vi "RobotGoToCoord.vi"(1 "X/Y/a Target":T11, 2 "RobotDriveDevRef":T1={"DevStatus"={"status"=FALSE, "code"=0, "source"=""}, "Motors[]"=[], "Square Inputs"=FALSE, "Max Output"=1.0}) -> (0 "Done?":bool)   [LabVIEW 2014]
uses:
  <vilib>/Rock Robotics/WPI/RobotDrive/WPI_RobotDriveDevRef.ctl
  <vilib>/Rock Robotics/WPI/MotorControl/WPI_MotorControlDeviceRef.ctl
  <vilib>/Rock Robotics/WPI/MotorControl/WPI_MotorControlType.ctl
  <vilib>/Rock Robotics/SystemInterfaces/Typedef/FPGA_TypedefDigitalModule.ctl
  <vilib>/Rock Robotics/SystemInterfaces/DIO/FPGA_DIOPWMChannel.ctl
  <vilib>/Rock Robotics/WPI/PWM/WPI_PWMDeadband.ctl
  <vilib>/Rock Robotics/WPI/CAN/Jaguar/SubVIs/WPI_CANJaguar_ControlMode.ctl
  <vilib>/Rock Robotics/WPI/CAN/TalonSRX/WPI_CANTalonSRX_APIControlMode.ctl
  <vilib>/Rock Robotics/WPI/PWM/WPI_PWMTransform_ConPane.ctl
  Robot Global Data.vi
  <vilib>/express/express arith-compare/Formula/XNode/ExpressFormulaBlockNode.xnode
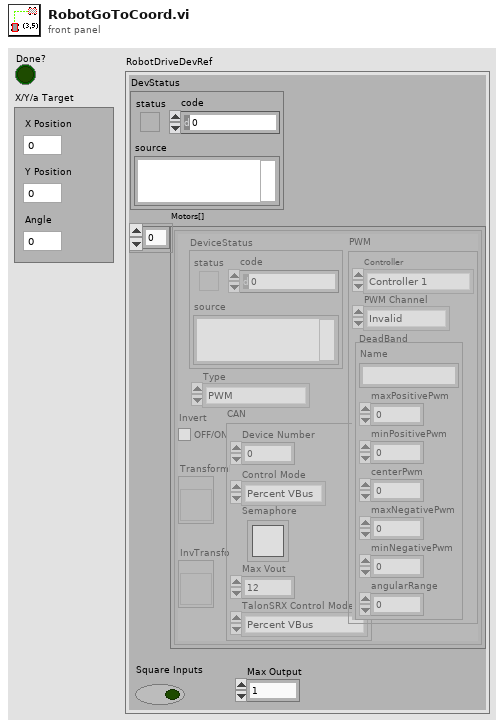
[diagram p1: front panel]
types:
  T1 = typedef "WPI_RobotDriveDevRef.ctl" = cluster{"DevStatus":errorcluster, "Motors[]":T2[], "Square Inputs":bool, "Max Output":dbl}
  T2 = typedef "WPI_MotorControlDeviceRef.ctl" = cluster{"DeviceStatus":errorcluster, "Type":T3, "PWM":cluster{"Controller":T4, "PWM Channel":T5, "DeadBand":T6}, "CAN":cluster{"Device Number":u8, "Control Mode":T7, "Semaphore":T8, "Max Vout":dbl, "TalonSRX Control Mode":T9}, "Invert":bool, "TransformRef":T10, "InvTransformRef":T10}
  T3 = typedef "WPI_MotorControlType.ctl" = enum16{"PWM", "CAN", "CANTalonSRX"}
  T4 = typedef "FPGA_TypedefDigitalModule.ctl" = enum16{"Controller 1"}
  T5 = typedef "FPGA_DIOPWMChannel.ctl" = enum8{"PWM 0", "PWM 1", "PWM 2", "PWM 3", "PWM 4", "PWM 5", "PWM 6", "PWM 7", "PWM 8", "PWM 9", "PWM MXP 0", "PWM MXP 1", "PWM MXP 2", "PWM MXP 3", "PWM MXP 4", "PWM MXP 5", "PWM MXP 6", "PWM MXP 7", "PWM MXP 8", "PWM MXP 9", "Invalid"}
  T6 = typedef "WPI_PWMDeadband.ctl" = cluster{"Name":string, "maxPositivePwm":i32, "minPositivePwm":i32, "centerPwm":i32, "maxNegativePwm":i32, "minNegativePwm":i32, "angularRange":u16}
  T7 = typedef "WPI_CANJaguar_ControlMode.ctl" = enum8{"Percent VBus", "Current", "Speed", "Position", "Voltage"}
  T8 = typedef "Semaphore RefNum" = refnum<k1>
  T9 = typedef "WPI_CANTalonSRX_APIControlMode.ctl" = enum8{"Percent VBus", "Speed", "Position", "Slave", "Unchanged / Invalid"}
  T10 = typedef "WPI_PWMTransform_ConPane.ctl" = refnum<vi>
  T11 = cluster{"X Position":dbl, "Y Position":dbl, "Angle":dbl}
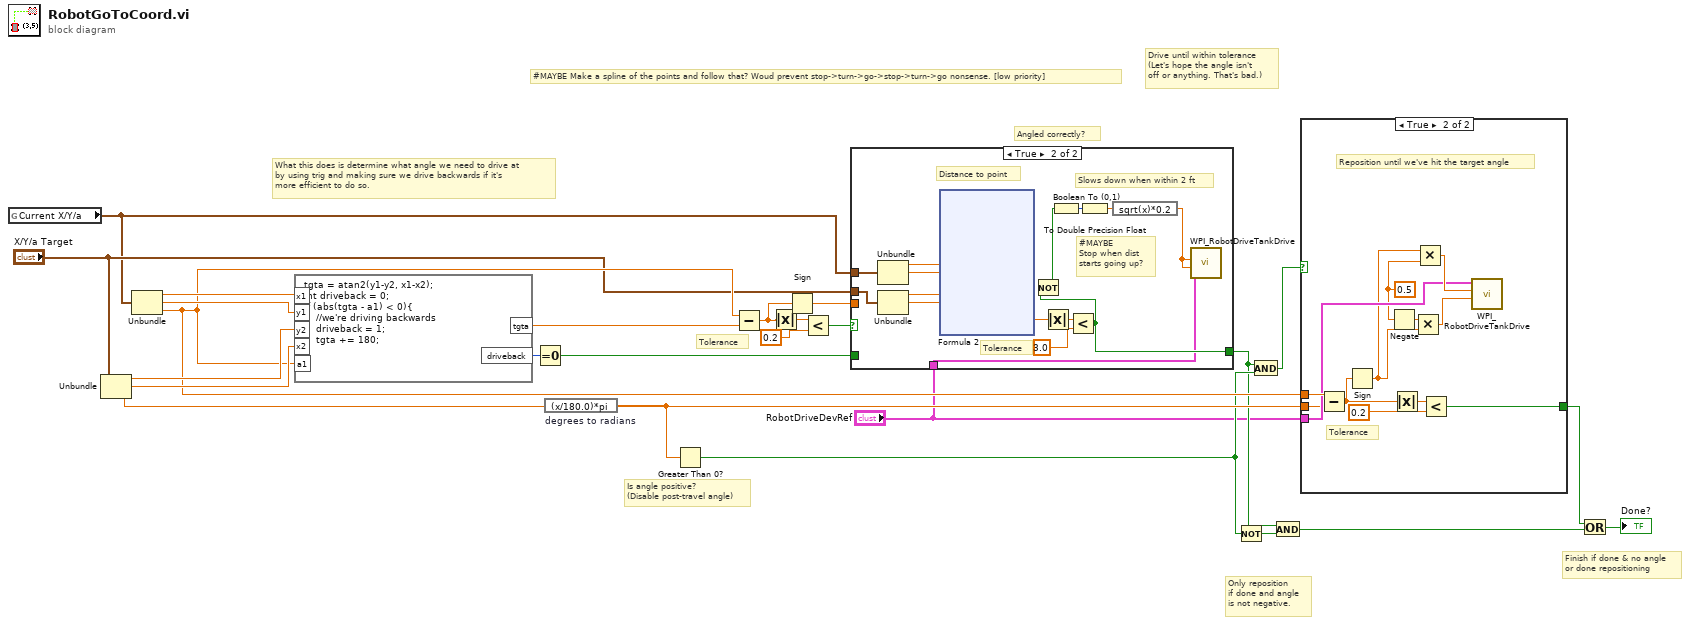
[diagram p0: block diagram]
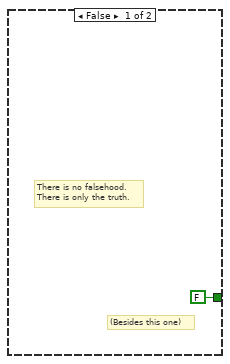
[diagram p2: hidden frame]
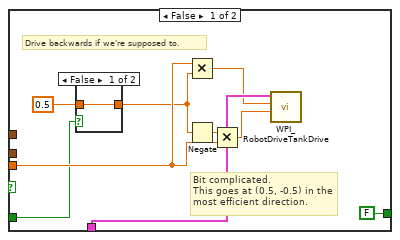
[diagram p3: hidden frame]
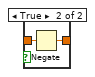
[diagram p4: hidden frame]
diagram:
  # "Drive until within tolerance\n(Let's hope the angle isn't\noff or anything. That's bad.)"
  # "What this does is determine what angle we need to drive at\nby using trig and making sure we drive backwards if it's\nmore efficient to do so."
  # "#MAYBE Make a spline of the points and follow that? Woud prevent stop->turn->go->stop->turn->go nonsense. [low priority]"
  # "Finish if done & no angle\nor done repositioning"
  # "Only reposition\nif done and angle\nis not negative."
  # "Is angle positive?\n(Disable post-travel angle)"
  # "Tolerance"
  # "Angled correctly?"
  n1 = global read "Robot Global Data.vi" "Current X/Y/a"() -> (w8:T11)
  n2 = Unbundle("X/Y/a Target") -> ("X Position"=w13:dbl, "Y Position"=w12:dbl, "Angle"=w18:dbl)
  n3 = Unbundle(w8) -> ("X Position"=w15:dbl, "Y Position"=w11:dbl, "Angle"=w10:dbl)
  n4 = formula code="tgta = atan2(y1-y2, x1-x2);\nint driveback = 0;\nif (abs(tgta - a1) < 0){\n    //we're driving backwards\n    driveback = 1;\n    tgta += 180;\n}"("x1"=w15, "y1"=w11, "y2"=w12, "x2"=w13, "a1"=w10) -> ("tgta"=w14:dbl, "driveback"=w7:i32)
  n5 = Equal To 0?(x=w7) -> (x = 0?=w6:bool)
  n6 = expression code="(x/180.0)*pi" "degrees to radians"(w18) -> (w17:dbl)
  n7 = Greater Than 0?(x=w17) -> (x > 0?=w5:bool)
  n8 = Subtract(x=w10, y=w14) -> (x-y=w22:dbl)
  n9 = Absolute Value(x=w22) -> (abs(x)=w21:dbl)
  n10 = Sign(1:w22) -> (0:w23:dbl)
  n11 = Less?(x=w21, y=0.2) -> (x < y?=w25:bool)
  n12 = case shown="True" w25 {
    tunnel: "RobotDriveDevRef" -> [w33 w40]
    tunnel: w23 -> [w29 _]
    tunnel: [FALSE w43] -> w3
    tunnel: "X/Y/a Target" -> [_ w50]
    tunnel: w8 -> [_ w47]
    tunnel: w6 -> [w28 _]
    frame False {
      # "Drive backwards if we're supposed to."
      # "Bit complicated.\nThis goes at (0.5, -0.5) in the most efficient direction."
      n13 = case shown="False" w28 {
        tunnel: 0.5 -> [w35 w37]
        tunnel: [w35 w36] -> w26
        frame False {
        }
        frame True {
          n14 = Negate(x=w37) -> (-x=w36:dbl)
        }
      }
      n15 = Multiply(x=w29, y=w26) -> (x*y=w32:dbl)
      n16 = Negate(x=w26) -> (-x=w34:dbl)
      n17 = Multiply(x=w34, y=w29) -> (x*y=w31:dbl)
      n18 = call <vilib>:"WPI_RobotDriveTankDrive.vi"("Right axis value"=w31, "Left axis value"=w32, "RobotDriveDevRef"=w33) -> ()  [unwired: 6 in, 3 out]
    }
    frame True {
      # "Slows down when within 2 ft"
      # "#MAYBE\nStop when dist\nstarts going up?"
      # "Tolerance"
      # "Distance to point"
      n19 = Unbundle(w47) -> ("X Position"=w46:dbl, "Y Position"=w45:dbl)  [unwired: 1 out]
      n20 = Unbundle(w50) -> ("X Position"=w49:dbl, "Y Position"=w48:dbl)  [unwired: 1 out]
      n21 = xnode "Formula 2"("X2"=w46, "Y2"=w45, "X1"=w49, "Y1"=w48) -> ("Result"=w44:dbl)  [unwired: 1 in, 1 out]
      n22 = Absolute Value(x=w44) -> (abs(x)=w51:dbl)
      n23 = Less?(x=w51, y=3.0) -> (x < y?=w43:bool)
      n24 = Not(x=w43) -> (.not. x?=w42:bool)
      n25 = Boolean To (0,1)(Boolean=w42) -> (0, 1=w41:i16)
      n26 = To Double Precision Float(number=w41) -> (double precision float=w39:dbl)
      n27 = expression code="sqrt(x)*0.2"(w39) -> (w38:dbl)
      n28 = call <vilib>:"WPI_RobotDriveTankDrive.vi"("Right axis value"=w38, "Left axis value"=w38, "RobotDriveDevRef"=w40) -> ()  [unwired: 6 in, 3 out]
    }
  }
  n29 = Not(x=w5) -> (.not. x?=w2:bool)
  n30 = And(x=w3, y=w5) -> (x .and. y?=w16:bool)
  n31 = And(x=w3, y=w2) -> (x .and. y?=w4:bool)
  n32 = case shown="True" w16 {
    tunnel: w10 -> [_ w78]
    tunnel: w17 -> [_ w70]
    tunnel: "RobotDriveDevRef" -> [_ w74]
    tunnel: [FALSE w73] -> w19
    frame False {
      # "(Besides this one)"
      # "There is no falsehood.\nThere is only the truth."
    }
    frame True {
      w68 = 0.5
      # "Reposition until we've hit the target angle"
      # "Tolerance"
      n33 = Subtract(x=w78, y=w70) -> (x-y=w71:dbl)
      n34 = Sign(1:w71) -> (0:w69:dbl)
      n35 = Negate(x=w68) -> (-x=w77:dbl)
      n36 = Absolute Value(x=w71) -> (abs(x)=w72:dbl)
      n37 = Multiply(x=w77, y=w69) -> (x*y=w75:dbl)
      n38 = Multiply(x=w69, y=w68) -> (x*y=w76:dbl)
      n39 = Less?(x=w72, y=0.2) -> (x < y?=w73:bool)
      n40 = call <vilib>:"WPI_RobotDriveTankDrive.vi"("Right axis value"=w75, "Left axis value"=w76, "RobotDriveDevRef"=w74) -> ()  [unwired: 6 in, 3 out]
    }
  }
  n41 = Or(x=w19, y=w4) -> (x .or. y?=→"Done?":bool)
